vi "GetRIAQtiveChannelNumber.vi"(2 "error in (no error)":errorcluster, 3 "Channel Settings":T1[](array[typedef])) -> (0 "error out":errorcluster, 1 "Numeric":i16)   [LabVIEW 2014]
doc: "Acquires total number of RIAQtive channels per given card. To be nested within a higher-level 'for' loop in order to access other cards. The numeric output of this VI determines the # of iterations the RIO channel storage VI will run."
uses:
  Controls/RIOSettingsChannelSettings.ctl
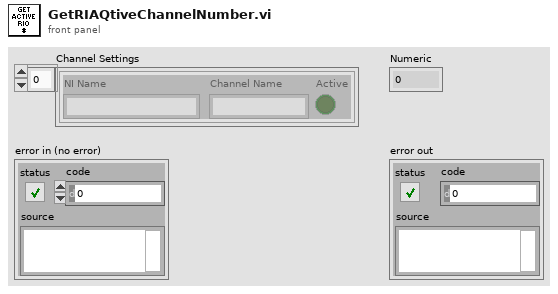
[diagram p1: front panel]
types:
  T1 = typedef "RIOSettingsChannelSettings.ctl" = cluster{"Channel Name":string, "Active":bool, "NI Name":string}
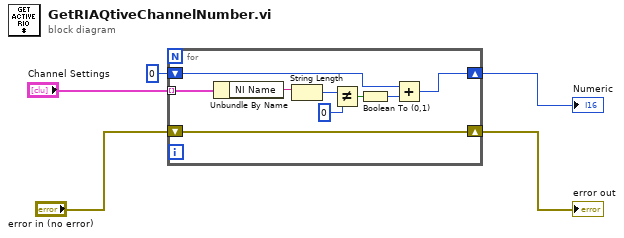
[diagram p0: block diagram]
diagram:
  n1 = for {
    tunnel: "Channel Settings" -> [w14] mode=indexing
    shift-right: [w13] -> w5
    shift-left: "error in (no error)" -> [w13]
    shift-right: [w6] -> w3
    shift-left: i16 0 -> [w7]
    n2 = Unbundle By Name(w14) -> ("NI Name"=w12:string)
    n3 = String Length(string=w12) -> (length=w10:i32)
    n4 = Not Equal?(x=w10, y=0) -> (x != y?=w9:bool)
    n5 = Boolean To (0,1)(Boolean=w9) -> (0, 1=w8:i16)
    n6 = Add(x=w7, y=w8) -> (x+y=w6:i16)
  }
  "error out" <- w5
  "Numeric" <- w3
